vi "Report_A131258.vi"(6 "文件重命名":bool, 7 "文件名称":string, 8 "错误输入（无错误）":errorcluster, 11 "布尔数组":bool[][](array[boolean])=[[TRUE]]) -> (0 "error out":errorcluster caption="错误输出", 3 "工件状态":string)   [LabVIEW 2020]
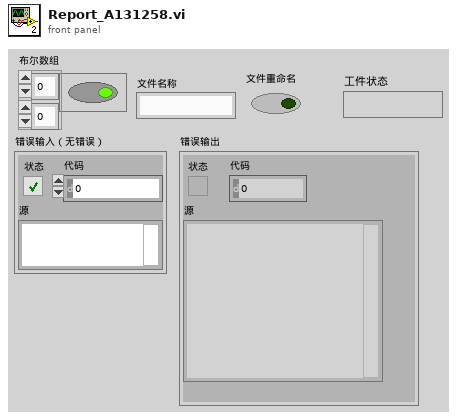
[diagram p1: front panel]
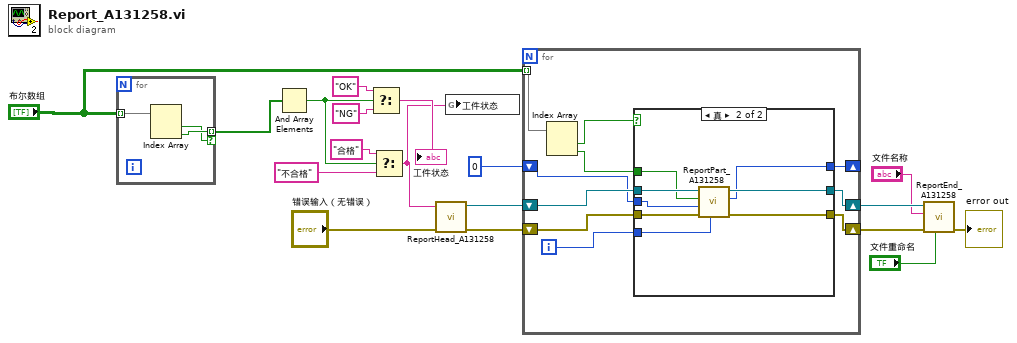
[diagram p0: block diagram]
diagram:
  n1 = for {
    tunnel: "布尔数组" -> [w21] mode=indexing
    tunnel: [w20] -> w4 mode=indexing if=w19
    n2 = Index Array(array=w21) -> (element #1=w19:bool, element #2=w20:bool)  [unwired: 2 in]
  }
  n3 = And Array Elements(Boolean array=w4) -> (logical AND=w6:bool)
  n4 = Select(t="OK", s=w6, f="NG") -> (s? t:f=→"工件状态":string)
  n5 = Select(t="合格", s=w6, f="不合格") -> (s? t:f=w1:string)
  n6 = call "ReportHead_A131258.vi"("error in (no error)"="错误输入（无错误）", "产品状态"=w1) -> ("error out"=w17:errorcluster, "report out"=w18:refnum<class "NI_report.lvclass">)  [unwired: 8 in]
  n7 = global write "追溯全部变量.vi" "工件状态"(w1) -> ()
  n8 = for {
    shift-right: [w29] -> w16
    shift-left: w18 -> [w31]
    shift-right: [w28] -> w15
    shift-left: w17 -> [w30]
    tunnel: "布尔数组" -> [w26] mode=indexing
    shift-right: [w22] -> _
    shift-left: 0 -> [w23]
    i -> [w27]
    n9 = Index Array(array=w26) -> (element #1=w25:bool, element #2=w24:bool)  [unwired: 2 in]
    n10 = case shown="真" w25 {
      tunnel: w31 -> [w33 w42]
      tunnel: w30 -> [w34 w41]
      tunnel: [w33 w40] -> w29
      tunnel: [w34 w39] -> w28
      tunnel: w27 -> [_ w37]
      tunnel: w24 -> [_ w38]
      tunnel: w23 -> [w32 w36]
      tunnel: [w32 w35] -> w22
      frame False {
      }
      frame True {
        n11 = call "ReportPart_A131258.vi"("试验项目"=w37, "error in"=w41, "索引"=w36, "合格"=w38, "report in"=w42) -> ("error out 2"=w39:errorcluster, "索引OUT"=w35:i32, "report out"=w40:refnum<class "NI_report.lvclass">)  [unwired: 4 in]
      }
    }
  }
  n12 = call "ReportEnd_A131258.vi"("文件重命名"="文件重命名", "error in (no error)"=w15, "文件名称"="文件名称", "report in"=w16) -> ("error out"=→"error out":errorcluster)  [unwired: 7 in]
